vi "test Expedited Download I32 C5-E.vi"(11 "Test Case In":refnum<class "Tests SDO Manager.lvclass">) -> (0 "error out":errorcluster, 3 "Test Case Out":refnum<class "Tests SDO Manager.lvclass">)   [LabVIEW 2020, in "Tests SDO Manager.lvclass"]
uses:
  Tests SDO Manager.lvclass
  C:/Program Files/National Instruments/LabVIEW 2026/vi.lib/Astemes/LUnit/Test Case.lvclass
  HAL/HAL-Devices/source/PCAN USB Dongle/PCAN Basic 4/Configure Strategies/Read-Write CAN Frame Strategy/PCAN Basic4 Read-Write CAN CC Frame Strategy.lvclass
  D:/git/HAL/Source/Interfaces/IApplyConfiguration/IApplyConfiguration.lvclass
  HAL/Source/Communicator/Communicator.lvclass
  D:/git/HAL/Source/Interfaces/ICommunicate/ICommunicate.lvclass
  source/Logging/Logger/Logger.lvclass
  C:/Program Files/National Instruments/LabVIEW 2026/vi.lib/ActorFramework/Actor/Actor.lvclass
  source/Logging/Logger/Logger.lvclass/Logger.ctl
  source/SDO Manager/SDO Manager/SDO Manager/SDO Manager.lvclass/SDO Manager.ctl
  <vilib>/ActorFramework/Message Enqueuer/Message Enqueuer.lvclass/Message Enqueuer.ctl
  <vilib>/Astemes/LUnit/Test Case.lvclass/Test Case.ctl
  <vilib>/ActorFramework/Stop Msg/Stop Msg.lvclass
  C:/Program Files/National Instruments/LabVIEW 2026/vi.lib/ActorFramework/Message/Message.lvclass
  HAL/Source/Interfaces/IMessage/IMessage.lvclass
  source/SDO Manager/SDO Manager/SDO Manager/SDO Manager.lvclass
  <vilib>/ActorFramework/Actor/Actor.lvclass
  source/Typedefs/Multiplexer.ctl
  source/CANopen.lvlib
  <vilib>/Astemes/LUnit/Test Case.lvclass
  source/Logging/Log Level.vi
  source/Logging/CANopen Logging.lvlib
  source/SDO Manager/SDO Manager/SDO Manager/Download I32.vi
  source/SDO Manager/SDO Manager/SDO Manager/Upload U32.vi
  source/SDO Manager/SDO Manager/SDO Transfer/SDO abort code.ctl
  source/SDO Manager/SDO Manager/SDO Transfer/SDO Transfer.lvclass
  source/Typedefs/SDO Result.ctl
panel:
  out "SDO Result":T1={"Success"=FALSE, "SDO abort code"={"Null"=TRUE, "Value"=84082688}, "Data"={"Null"=TRUE, "Data"=[]}} {"SDO abort code"."Value" items=["Toggle bit not allowed"=84082688, "SDO protocol timed out"=84148224, "Client/server command specifier not valid or unknown"=84148225, "Invalid block size (block mode only)"=84148226, "Invalid sequence number (block mode only)"=84148227, "CRC error (block mode only)"=84148228, "Out of memory"=84148229, "Attempt to read a write only object"=100728833, "Attempt to write a read only object"=100728834, "Object does not exist in the object dictionary"=100794368, "Object cannot be mapped to the PDO"=100925505, "The number and length of the objects to be mapped would exceed PDO length"=100925506, "General parameter incompatibility reason"=100925507, "General internal incompatibility in the device"=100925511, "Access failed due to an hardware error"=101056512, "Data type does not match, length of service parameter does not match"=101122064, "Data type does not match, length of service parameter too high"=101122066, "Data type does not match, length of service parameter too low"=101122067, "Sub-index does not exist"=101253137, "Invalid value for parameter (download only)"=101253168, "Value of parameter written too high (download only)"=101253169, "Value of parameter written too low (download only)"=101253170, "Maximum value is less than minimum value"=101253174, "Resource not available: SDO connection"=101318691, "General error"=134217728, "Data cannot be transferred or stored to the application"=134217760, "Data cannot be transferred or stored to the application because of local control"=134217761, "Data cannot be transferred or stored to the application because of the present device stable"=134217762, "Object dictionary dynamic generation fails or no object dictionary is present (e.g. object dictionary is generated from file and generation fails because of an file error)"=134217763, "No data available"=134217764]; "Data"."Data" format="%02x"}
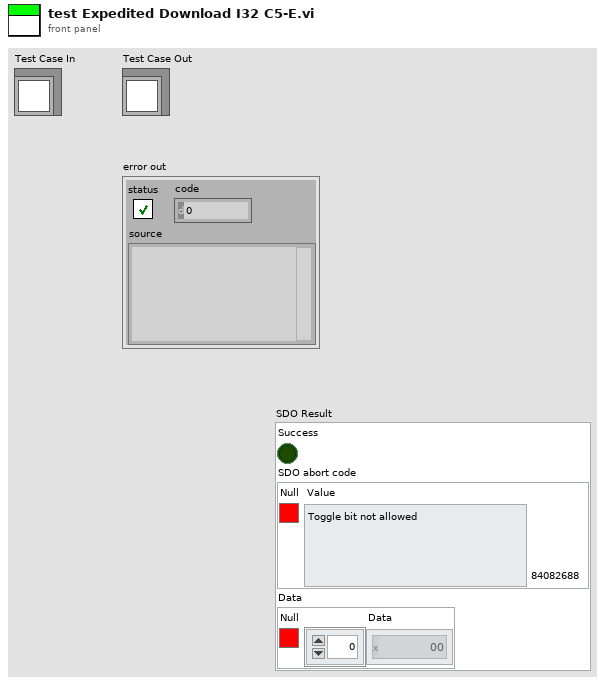
[diagram p1: front panel]
types:
  T1 = typedef "CANopen.lvlib/SDO Manager.lvlib/SDO Transfer.lvclass/SDO Result.ctl" = cluster{"Success":bool, "SDO abort code":cluster{"Null":bool, "Value":T2}, "Data":cluster{"Null":bool, "Data":u8[]}}
  T2 = typedef "CANopen.lvlib/SDO Manager.lvlib/SDO Transfer.lvclass/SDO abort code.ctl" = u32
  T3 = typedef "CANopen.lvlib/Multiplexer.ctl" = cluster{"Index":u16, "Sub Index":u8}
  T4 = enum16{"Error", "Warn", "Info", "Debug", "Trace"}
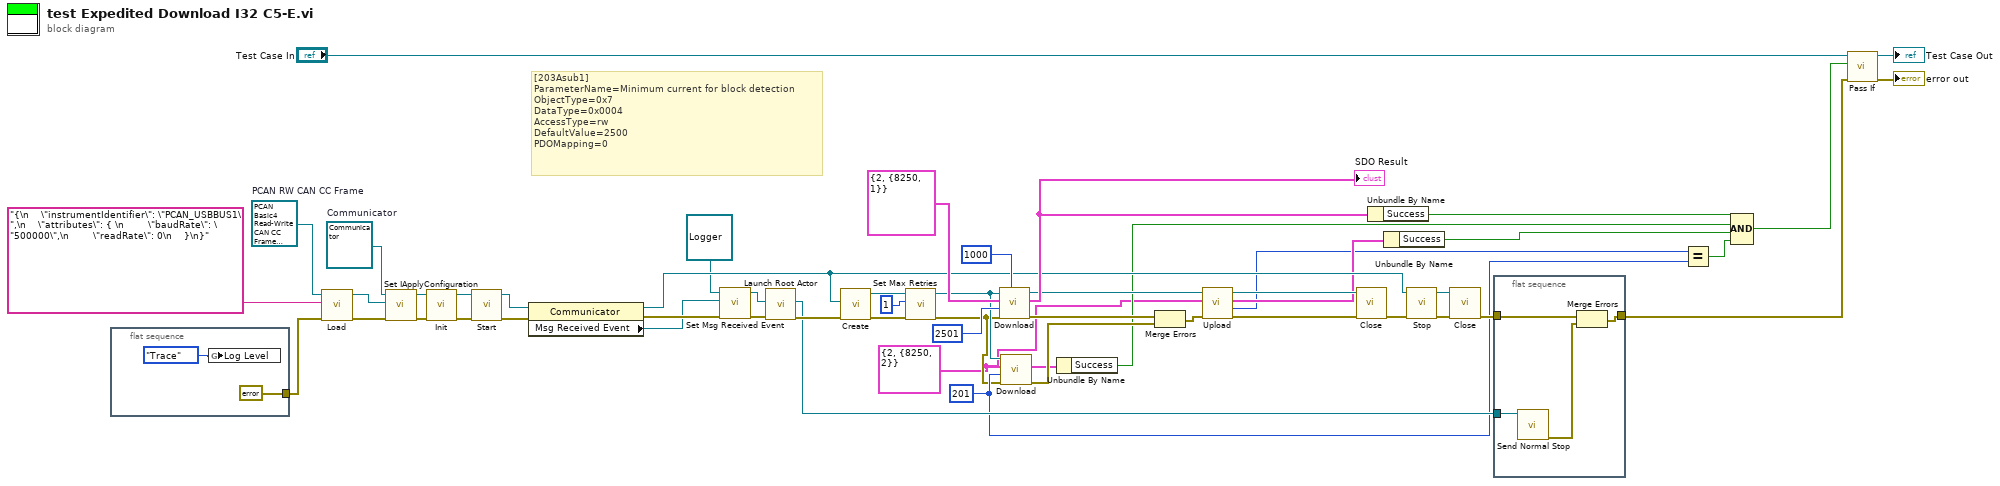
[diagram p0: block diagram]
diagram:
  w3 = 201 ("Value")
  w1 = cluster{"Node-ID":u8, "Multiplexer":T3} {"Node-ID"=2, "Multiplexer"={"Index"=8250, "Sub Index"=2}} ("Parameters")
  w28 = refnum<class "Communicator.lvclass"> refnum  # Communicator
  w35 = refnum<class "PCAN Basic4 Read-Write CAN CC Frame Strategy.lvclass"> refnum  # PCAN RW CAN CC Frame
  # "[203Asub1]\nParameterName=Minimum current for block detection\nObjectType=0x7\nDataType=0x0004\nAccessType=rw\nDefaultValue=2500\nPDOMapping=0"
  n1 = flat-sequence {
    tunnel: [errorcluster {"status"=FALSE, "code"=0, "source"=""} ("error constant")] -> w33
    frame #0 {
      n2 = global write "Log Level.vi" "Log Level"(T4."Trace" ("Log Level")) -> ()
    }
  }
  n3 = call-dynamic "Load.vi"("error in"=w33, "Source"="{\n    \"instrumentIdentifier\": \"PCAN_USBBUS1\",\n    \"attributes\": { \n        \"baudRate\": \"500000\",\n        \"readRate\": 0\n    }\n}", "PCAN Basic Base Configure Strategy in"=w35) -> ("error out"=w31:errorcluster, "PCAN Basic Base Configure Strategy out"=w32:refnum<class "PCAN Basic4 Read-Write CAN CC Frame Strategy.lvclass">)  [unwired: 7 in]
  n4 = call-dynamic "Set IApplyConfiguration.vi"("Error In"=w31, "IApplyConfiguration"=w32, "Communicator in"=w28) -> ("Error Out"=w30:errorcluster, "Communicator out"=w29:refnum<class "Communicator.lvclass">)  [unwired: 7 in]
  n5 = call-dynamic "Init.vi"("Error In"=w30, "Communicator in"=w29) -> ("Error Out"=w27:errorcluster, "Communicator out"=w26:refnum<class "Communicator.lvclass">)  [unwired: 8 in]
  n6 = call-dynamic "Start.vi"("Error In"=w27, "Communicator in"=w26) -> ("Error Out"=w25:errorcluster, "Communicator out"=w24:refnum<class "Communicator.lvclass">)  [unwired: 8 in]
  n7 = property class="Communicator"(reference=w24, error in=w25) -> (reference out=w21:refnum<class "Communicator.lvclass">, error out=w44:errorcluster, "Msg Received Event"=w20:refnum<user-event>)
  n8 = call "Set Msg Received Event.vi"("error in"=w44, "Msg Received Event"=w20, "Logger in"=refnum<class "Logger.lvclass"> refnum) -> ("error out"=w46:errorcluster, "Logger out"=w45:refnum<class "Logger.lvclass">)  [unwired: 7 in]
  n9 = call <vilib>:"Launch Root Actor.vi"("error in (no error)"=w46, "Actor"=w45) -> ("error out"=w19:errorcluster, "Actor's Enqueuer"=w18:refnum<class "Message Enqueuer.lvclass">)  [unwired: 8 in]
  n10 = call "Create.vi"("Error In"=w19, "ICommunicate"=w21) -> ("Error Out"=w41:errorcluster, "SDO Manager"=w40:refnum<class "SDO Manager.lvclass">)  [unwired: 8 in]
  n11 = call "Set Max Retries.vi"("error in"=w41, "Max Retries"=u8 1, "SDO Manager in"=w40) -> ("error out"=w2:errorcluster, "SDO Manager out"=w16:refnum<class "SDO Manager.lvclass">)  [unwired: 7 in]
  n12 = call-poly "Download.vi"("Timeout"=1000, "error in"=w2, "Value"=u32 2501, "Parameters"=cluster{"Node-ID":u8, "Multiplexer":T3} {"Node-ID"=2, "Multiplexer"={"Index"=8250, "Sub Index"=1}}, "SDO Manager in"=w16) -> ("error out"=w48:errorcluster, "SDO Result"=w47:T1, "SDO Manager out"=w14:refnum<class "SDO Manager.lvclass">)  [unwired: 4 in]
  "SDO Result" <- w47
  n13 = call-poly "Download.vi"("error in"=w2, "Value"=w3, "Parameters"=w1, "SDO Manager in"=w16) -> ("error out"=w11:errorcluster, "SDO Result"=w10:T1)  [unwired: 5 in, 1 out]
  n14 = Unbundle By Name(w10) -> ("Success"=w8:bool)
  n15 = Merge Errors(w48, w11) -> (w12:errorcluster)
  n16 = call-poly "Upload.vi"("Error In"=w12, "Parameters"=w1, "SDO Manager in"=w14) -> ("Error Out"=w15:errorcluster, "Value"=w4:u32, "SDO Result"=w7:T1, "SDO Manager out"=w13:refnum<class "SDO Manager.lvclass">)  [unwired: 5 in]
  n17 = call "Close.vi"("Error In"=w15, "SDO Manager"=w13) -> ("Error Out"=w50:errorcluster)  [unwired: 8 in, 1 out]
  n18 = Unbundle By Name(w47) -> ("Success"=w38:bool)
  n19 = Unbundle By Name(w7) -> ("Success"=w6:bool)
  n20 = call-dynamic "Stop.vi"("Error In"=w50, "Communicator in"=w21) -> ("Error Out"=w23:errorcluster, "Communicator out"=w22:refnum<class "Communicator.lvclass">)  [unwired: 8 in]
  n21 = call-dynamic "Close.vi"("Error In"=w23, "Communicator in"=w22) -> ("Error Out"=w43:errorcluster)  [unwired: 8 in, 1 out]
  n22 = flat-sequence {
    tunnel: w43 -> [w58]
    tunnel: [w59] -> w42
    tunnel: w18 -> [w57]
    frame #0 {
      n23 = call <vilib>:"Send Normal Stop.vi"("Message Enqueuer"=w57) -> ("error out"=w56:errorcluster)  [unwired: 10 in]
      n24 = Merge Errors(w58, w56) -> (w59:errorcluster)
    }
  }
  n25 = Equal?(x=w4, y=w3) -> (x = y?=w5:bool)
  n26 = Compound Arithmetic op=AND(w38, w8, w6, w5) -> (w9:bool)
  n27 = call <vilib>:"Pass If.vi"("error in (no error)"=w42, "Pass?"=w9, "LUnit Test Case In"="Test Case In") -> ("error out"=→"error out":errorcluster, "LUnit Test Case Out"=→"Test Case Out":refnum<class "Tests SDO Manager.lvclass">)  [unwired: 7 in]
